vi "TargetCorner_New.vi"(9 "Y":dbl, 11 "X":dbl) -> (3 "TargetCorner":T1)   [LabVIEW 2019, in "PhotonVisionLib.lvlib"]
doc: "Create a new TargetCorner data cluster\n\nInputs:\n - X -- \n - Y -- \n\nOutputs:\n - TargetCorner -- Created TargetCorner cluster."
uses:
  PhotonVisionLib.lvlib
  TypeDef/TargetCornerType.ctl
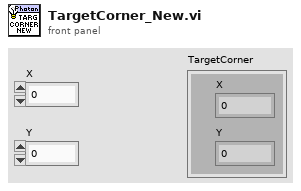
[diagram p1: front panel]
types:
  T1 = typedef "PhotonVisionLib.lvlib/TargetCornerType.ctl" = cluster{"X":dbl, "Y":dbl}
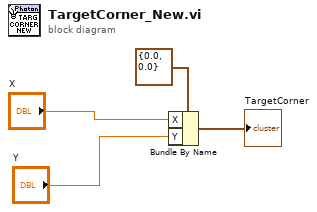
[diagram p0: block diagram]
diagram:
  n1 = Bundle By Name(cluster=T1 {"X"=0.0, "Y"=0.0} ("TargetCorner"), "X"="X", "Y"="Y") -> (→"TargetCorner":T1)
